vi "Global Data.vi"() -> ()   [LabVIEW 2015]
panel:
  out "teamNumberChange":bool
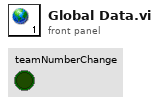
[diagram p1: front panel]
diagram:
